vi "Parse String.vi"(8 "Error In":errorcluster, 9 "JSON Response":string, 10 "Key":string, 11 "XBMC Ref":T1={"HTTP Handle"=refnum, "Hostname / IP"="localhost", "jsonrpc"="2.0"}) -> (0 "Error Out":errorcluster, 1 "Dup JSON Response":string, 2 "Value":string, 3 "XBMC Ref":T1={"HTTP Handle"=refnum, "Hostname / IP"="localhost", "jsonrpc"="2.0"})   [LabVIEW 2013, in "LMH-Kodi.lvlib"]
uses:
  LMH-Kodi.lvlib
  Type Defs/XBMC Ref.ctl
  <vilib>/httpClient/ClientHandle.ctl
  <vilib>/httpClient/LabVIEWHTTPClient.lvlib
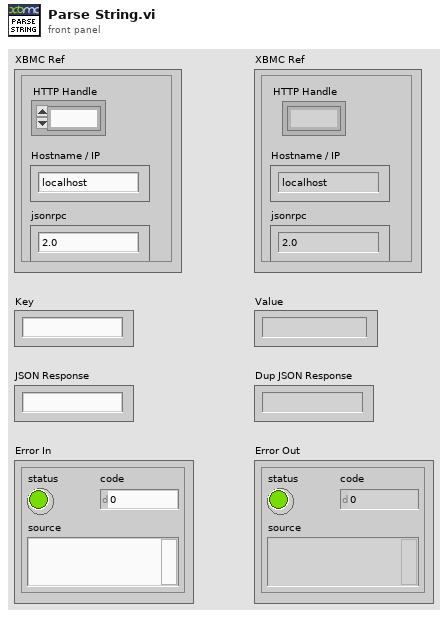
[diagram p1: front panel]
types:
  T1 = typedef "LMH-Kodi.lvlib/XBMC Ref.ctl" = cluster{"HTTP Handle":T2, "Hostname / IP":string, "jsonrpc":string}
  T2 = typedef "LabVIEWHTTPClient.lvlib/ClientHandle.ctl" = refnum<k1>
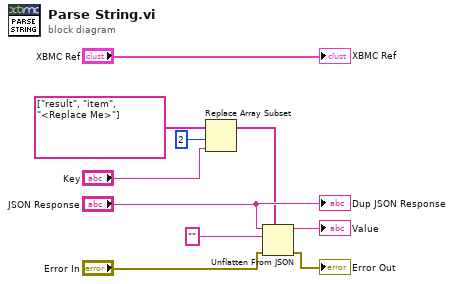
[diagram p0: block diagram]
diagram:
  n1 = Replace Array Subset(array=string[] ["result", "item", "<Replace Me>"] ("path"), new element="Key", index=2) -> (w5:string[])
  n2 = Unflatten From JSON(path=w5, JSON string="JSON Response", type and defaults="", error in (no error)="Error In") -> (value=→"Value":string, error out=→"Error Out":errorcluster)  [unwired: 3 in]
  "Dup JSON Response" <- "JSON Response"
  "XBMC Ref" <- "XBMC Ref"
